vi "SSL Read.vi"(6 "IPCS ?":bool, 7 "Buffer Size":i32=1024, 8 "Error In":errorcluster, 11 "SSL Stream":refnum<k24>) -> (0 "Error Out":errorcluster, 2 "Message Read":string, 4 "Client Connected ?":bool)   [LabVIEW 2014, in "SSL Lib.lvlib"]
doc: "VI Function: This VI reads the data from client over the SSL stream.\n\nVI Version: 1.0\n\nVI Author: Runjhun Agarwal"
uses:
  <userlib>/SSL Library/SSL Lib.lvlib
panel:
  out "CanRead":bool
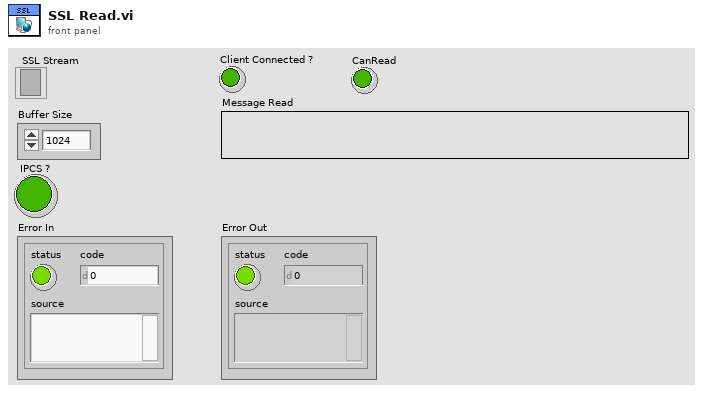
[diagram p1: front panel]
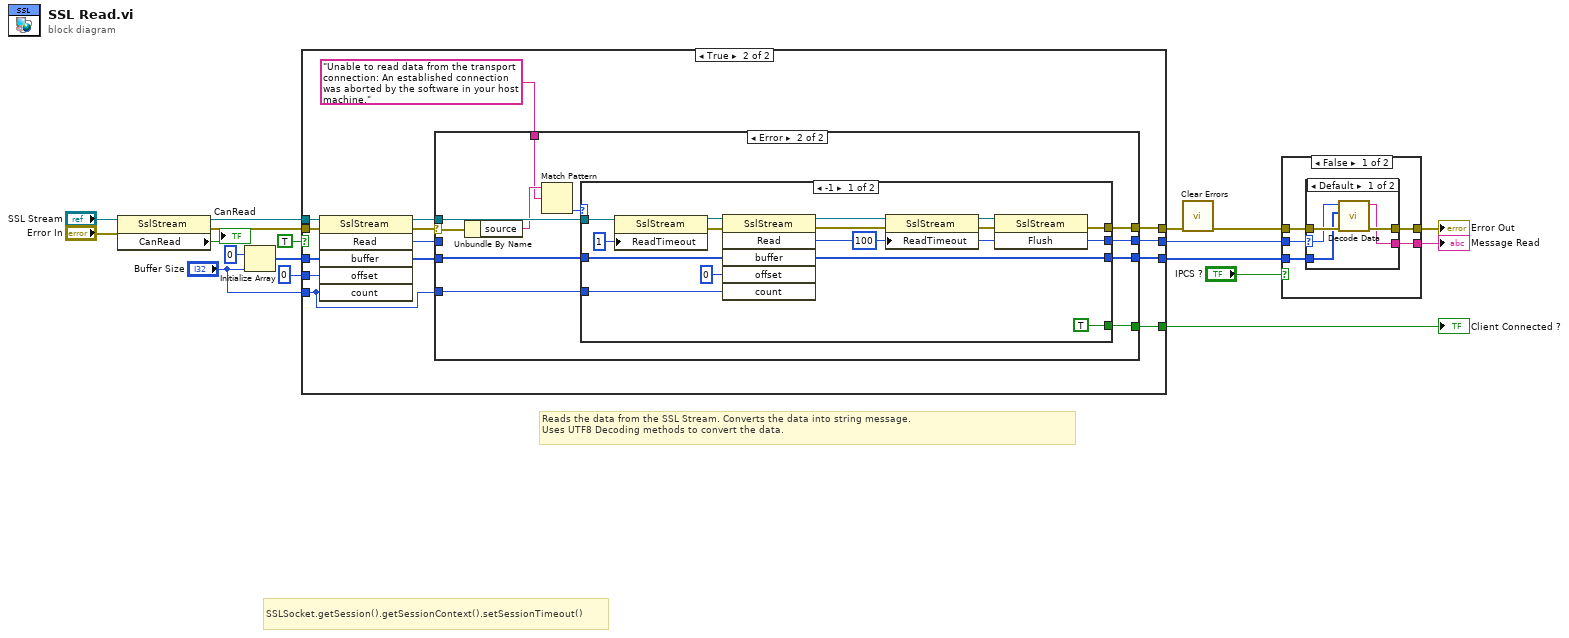
[diagram p0: block diagram]
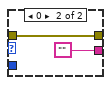
[diagram p2: hidden frame]
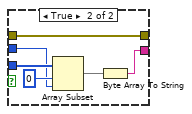
[diagram p3: hidden frame]
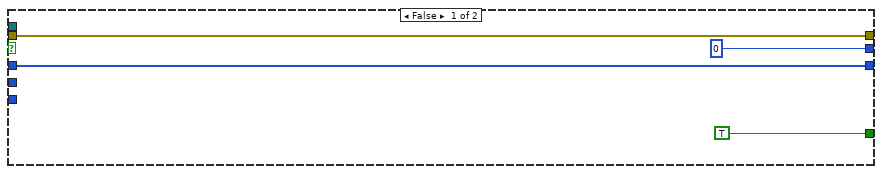
[diagram p4: hidden frame]
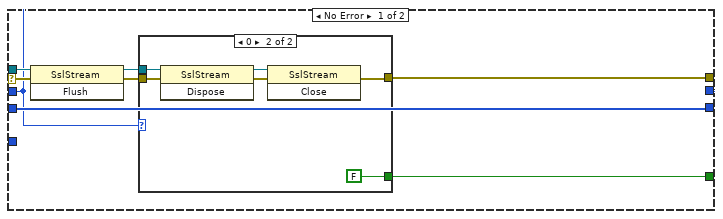
[diagram p5: hidden frame]
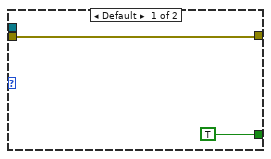
[diagram p6: hidden frame]
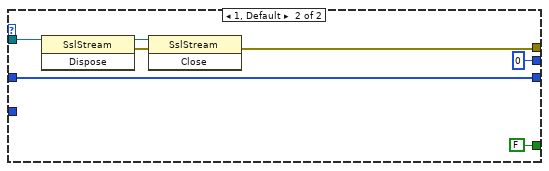
[diagram p7: hidden frame]
diagram:
  # "SSLSocket.getSession().getSessionContext().setSessionTimeout()"
  # "Reads the data from the SSL Stream. Converts the data into string message.\nUses UTF8 Decoding methods to convert the data."
  n1 = property class="SslStream"(reference="SSL Stream", error in="Error In") -> (reference out=w11:refnum<k24>, error out=w10:errorcluster, "CanRead"=→"CanRead":bool)
  n2 = Initialize Array(u8 0 ("element"), "Buffer Size") -> (w17:u8[])
  n3 = case shown="True" TRUE {
    tunnel: 0 ("offset") -> [_ w24]
    tunnel: w17 -> [w20 w25]
    tunnel: "Buffer Size" -> [_ w23]
    tunnel: [w22 w30] -> w9
    tunnel: [w20 w32] -> w13
    tunnel: [0 ("Read") w31] -> w12
    tunnel: w11 -> [_ w36]
    tunnel: w10 -> [w22 w35]
    tunnel: [TRUE w27] -> w1
    frame False {
    }
    frame True {
      n4 = invoke class="SslStream" method="Read"(reference=w36, error in=w35, "buffer"=w25, "offset"=w24, "count"=w23) -> (reference out=w33:refnum<k24>, error out=w34:errorcluster, "Read"=w29:i32, "buffer"=w26:u8[])  [unwired: 1 in, 2 out]
      n5 = case shown="Error" w34 {
        selector: w34 -> [w43 w57]
        tunnel: w33 -> [w42 w63]
        tunnel: w26 -> [w44 w62]
        tunnel: w23 -> [_ w61]
        tunnel: [w44 w60] -> w32
        tunnel: [w41 w59] -> w31
        tunnel: [w39 w58] -> w30
        tunnel: w29 -> [w41 _]
        tunnel: "Unable to read data from the transport connection: An established connection was aborted by the software in your host machine." -> [_ w55]
        tunnel: [w37 w53] -> w27
        frame No Error {
          n6 = invoke class="SslStream" method="Flush"(reference=w42, error in=w43) -> (reference out=w38:refnum<k24>, error out=w40:errorcluster)  [unwired: 1 in, 1 out]
          n7 = case shown="0" w41 {
            tunnel: w40 -> [w46 w50]
            tunnel: [w46 w47] -> w39
            tunnel: w38 -> [_ w49]
            tunnel: [TRUE FALSE] -> w37
            frame Default {
            }
            frame 0 {
              n8 = invoke class="SslStream" method="Dispose"(reference=w49, error in=w50) -> (reference out=w51:refnum<k24>, error out=w52:errorcluster)  [unwired: 1 in, 1 out]
              n9 = invoke class="SslStream" method="Close"(reference=w51, error in=w52) -> (error out=w47:errorcluster)  [unwired: 1 in, 2 out]
            }
          }
        }
        frame Error {
          n10 = Unbundle By Name(w57) -> ("source"=w56:string)
          n11 = Match Pattern(string=w56, regular expression=w55) -> (offset past match=w54:i32)  [unwired: 1 in, 3 out]
          n12 = case shown="-1" w54 {
            tunnel: w63 -> [w79 w86]
            tunnel: w62 -> [w75 w82]
            tunnel: w61 -> [w73 _]
            tunnel: [w72 w82] -> w60
            tunnel: [w71 0 ("Read")] -> w59
            tunnel: [w65 w80] -> w58
            tunnel: [TRUE FALSE] -> w53
            frame -1 {
              n13 = property class="SslStream"(reference=w79, "ReadTimeout"=1) -> (reference out=w76:refnum<k24>, error out=w77:errorcluster)  [unwired: 1 in]
              n14 = invoke class="SslStream" method="Read"(reference=w76, error in=w77, "buffer"=w75, "offset"=0, "count"=w73) -> (reference out=w70:refnum<k24>, error out=w69:errorcluster, "Read"=w71:i32, "buffer"=w72:u8[])  [unwired: 1 in, 2 out]
              n15 = property class="SslStream"(reference=w70, error in=w69, "ReadTimeout"=100) -> (reference out=w67:refnum<k24>, error out=w66:errorcluster)
              n16 = invoke class="SslStream" method="Flush"(reference=w67, error in=w66) -> (error out=w65:errorcluster)  [unwired: 1 in, 2 out]
            }
            frame 1, Default {
              n17 = invoke class="SslStream" method="Dispose"(reference=w86) -> (reference out=w83:refnum<k24>, error out=w84:errorcluster)  [unwired: 2 in, 1 out]
              n18 = invoke class="SslStream" method="Close"(reference=w83, error in=w84) -> (error out=w80:errorcluster)  [unwired: 1 in, 2 out]
            }
          }
        }
      }
    }
  }
  "Client Connected ?" <- w1
  n19 = call <vilib>:"Clear Errors.vi"("error in (no error)"=w9) -> ("error out"=w14:errorcluster)  [unwired: 5 in, 1 out]
  n20 = case shown="False" "IPCS ?" {
    tunnel: [w91 w104] -> w15
    tunnel: w14 -> [w90 w104]
    tunnel: w13 -> [w89 w103]
    tunnel: w12 -> [w88 w101]
    tunnel: [w87 w99] -> w3
    frame False {
      n21 = case shown="Default" w88 {
        selector: w88 -> [w93 _]
        tunnel: [w94 ""] -> w87
        tunnel: [w95 w98] -> w91
        tunnel: w90 -> [w96 w98]
        tunnel: w89 -> [w92 _]
        frame Default {
          n22 = call <userlib>:"Decode Data.vi"("Error In"=w96, "Buffer"=w92, "Read"=w93) -> ("Error Out"=w95:errorcluster, "ToString"=w94:string)  [unwired: 7 in]
        }
        frame 0 {
        }
      }
    }
    frame True {
      n23 = Array Subset(array=w103, index=0, length=w101) -> (w100:u8[])
      n24 = Byte Array To String(unsigned byte array=w100) -> (string=w99:string)
    }
  }
  "Message Read" <- w3
  "Error Out" <- w15
